vi "Global Conveyor.vi"() -> ()   [LabVIEW 2019, in "Untitled Library 1.lvlib"]
uses:
  Untitled Library 1.lvlib
panel:
  in  "Shoot":bool
  in  "Climb Piston":bool
  in  "Spin Roulette":bool
  in  "Roulette":bool
  in  "Climb":bool
  in  "Disable Auto":bool
  in  "Intake":bool
  in  "Spin":bool
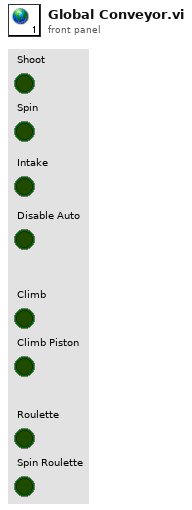
[diagram p1: front panel]
diagram:
